vi "Read Test Info.vi"(8 "error in (no error)":errorcluster, 11 "Refnum in":T1) -> (0 "error out":errorcluster, 3 "Test Details":string[](array[string]))   [LabVIEW 2017]
uses:
  <vilib>/addons/database/Connection.llb/Conn ObjectReference.ctl
  <vilib>/addons/database/NI_Database_API.lvlib
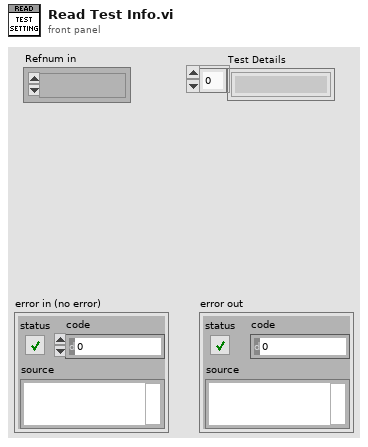
[diagram p1: front panel]
types:
  T1 = typedef "NI_Database_API.lvlib/Conn ObjectReference.ctl" = refnum<k1>
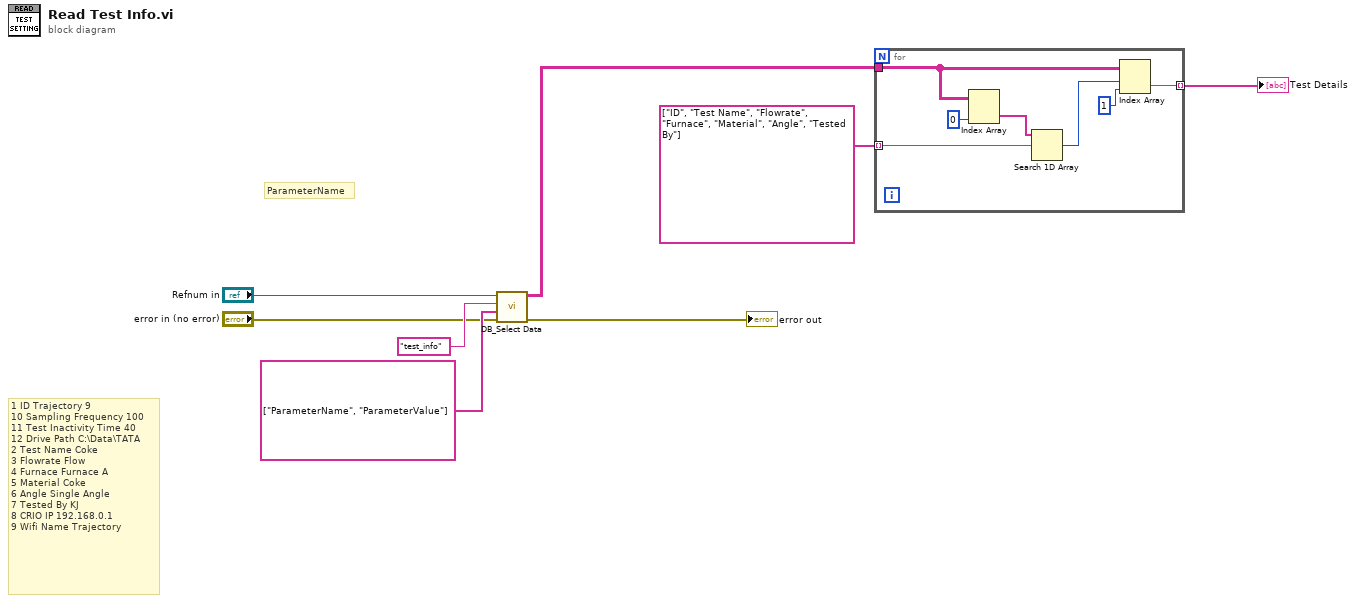
[diagram p0: block diagram]
diagram:
  # "ParameterName"
  # "1\tID\tTrajectory 9\n10\tSampling Frequency\t100\n11\tTest Inactivity Time\t40\n12\tDrive Path\tC:\\Data\\TATA\n2\tTest Name\tCoke\n3\tFlowrate\tFlow\n4\tFurnace\tFurnace A\n5\tMaterial\tCoke\n6\tAngle\tSingle Angle\n7\tTested By\tKJ\n8\tCRIO IP\t192.168.0.1\n9\tWifi Name\tTrajectory"
  n1 = call "DB_Select Data.vi"("error in (no error)"="error in (no error)", "columns"=string[] ["ParameterName", "ParameterValue"], "table"="test_info", "connection reference"="Refnum in") -> ("error out"=→"error out":errorcluster, "data"=w2:string[][])  [unwired: 6 in]
  n2 = for {
    tunnel: w2 -> [w12]
    tunnel: string[] ["ID", "Test Name", "Flowrate", "Furnace", "Material", "Angle", "Tested By"] ("columns") -> [w13] mode=indexing
    tunnel: [w9] -> w3 mode=indexing
    n3 = Index Array(array=w12, index (col)=0 ("disabled index (col)")) -> (element=w14:string[])  [unwired: 1 in]
    n4 = Search 1D Array(1D array=w14, element=w13) -> (index of element=w10:i32)  [unwired: 1 in]
    n5 = Index Array(array=w12, index (row)=w10, index (col)=1 ("disabled index (col)")) -> (element=w9:string)
  }
  "Test Details" <- w3
